vi "Get EST Lib Version from Bitfile.vi"(8 "error in (no error)":errorcluster, 11 "vi info":T2 {"RegisterMap"."Address" format="%.0x"}) -> (0 "error out":errorcluster, 1 "valid bitfile":bool, 2 "EST version enum":T1, 3 "vi info dup":T2 {"RegisterMap"."Address" format="%.0x"}, 5 "EST version string":string)   [LabVIEW 2020, in "Engine Simulation Toolkit System Explorer.lvlib"]
uses:
  Engine Simulation Toolkit System Explorer.lvlib
  <vilib>/rvi/Bitfile/niFpgaBitfileStructure_VI.ctl
  <vilib>/rvi/Bitfile/nirviControlStructure.ctl
  <vilib>/rvi/Bitfile/nirviTypdefDescription.ctl
  <vilib>/rvi/Bitfile/nirviMechanicalAction.ctl
  <vilib>/rvi/Bitfile/nirviSubControlStructure.ctl
  <vilib>/rvi/Bitfile/nirviClusterElementControl.ctl
  <vilib>/picture/picture.llb/imagedata.ctl
  Shared/Bitfile EST Version.ctl
  <vilib>/Utility/Data Type/NI_Data Type.lvlib
  Shared/Engine Simulation Toolkit Shared.lvlib
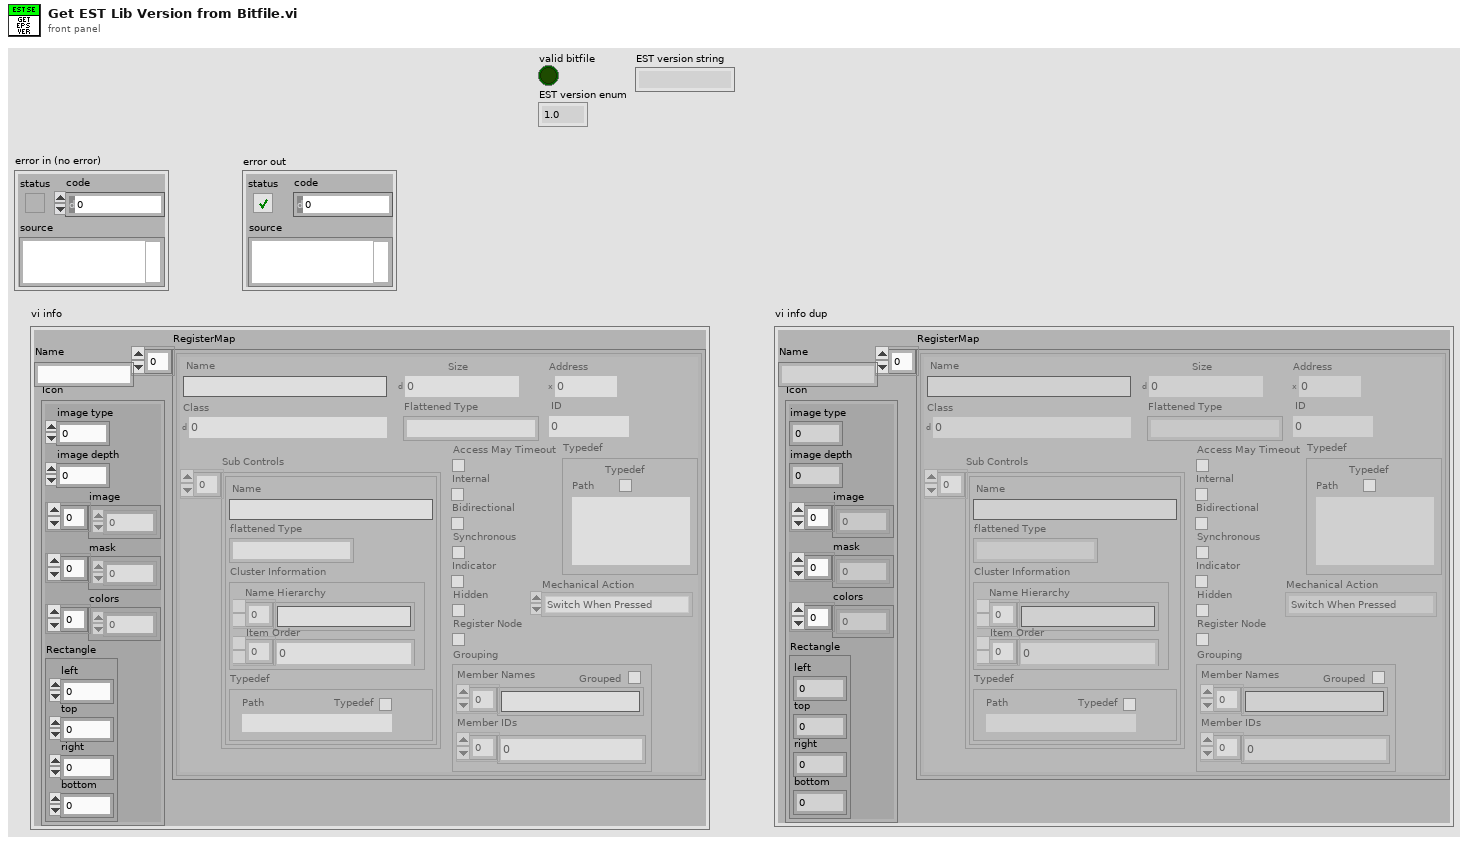
[diagram p1: front panel]
types:
  T1 = typedef "Engine Simulation Toolkit Shared.lvlib/Bitfile EST Version.ctl" = enum16{"1.0", "1.1", "1.2", "1.3", "1.4"}
  T2 = typedef "niFpgaBitfileStructure_VI.ctl" = cluster{"Name":string, "RegisterMap":T3[], "Icon":T8}
  T3 = typedef "nirviControlStructure.ctl" = cluster{"Name":string, "Hidden":bool, "Indicator":bool, "Flattened Type":string, "Grouping":cluster{"Grouped":bool, "Member Names":string[], "Member IDs":u32[]}, "Address":u32, "Size":u32, "Class":u32, "Internal":bool, "Typedef":T4, "ID":u32, "Bidirectional":bool, "Synchronous":bool, "Mechanical Action":T5, "Sub Controls":T6[], "Access May Timeout":bool, "Register Node":bool}
  T4 = typedef "nirviTypdefDescription.ctl" = cluster{"Typedef":bool, "Path":path}
  T5 = typedef "nirviMechanicalAction.ctl" = enum8{"Switch When Pressed", "Switch When Released", "Switch Until Released", "Latch When Pressed", "Latch When Released", "Latch Until Released"}
  T6 = typedef "nirviSubControlStructure.ctl" = cluster{"Name":string, "flattened Type":string, "Cluster Information":T7, "Typedef":T4}
  T7 = typedef "nirviClusterElementControl.ctl" = cluster{"Name Hierarchy":string[], "Item Order":u32[]}
  T8 = typedef "imagedata.ctl" = cluster{"image type":i32, "image depth":i32, "image":u8[], "mask":u8[], "colors":u32[], "Rectangle":cluster{"left":i16, "top":i16, "right":i16, "bottom":i16}}
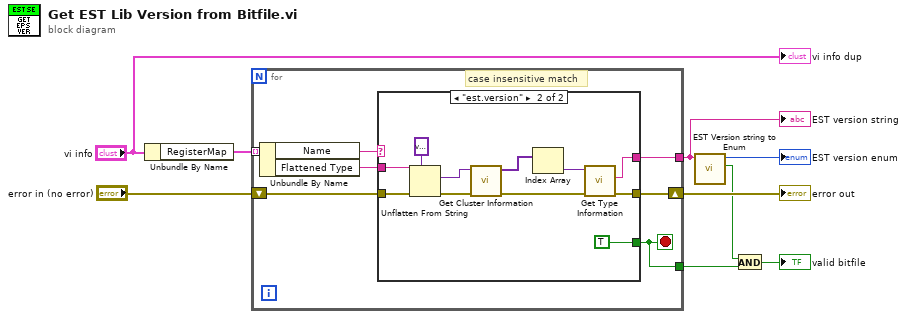
[diagram p0: block diagram]
diagram:
  n1 = Unbundle By Name("vi info") -> ("RegisterMap"=w8:T3[])
  n2 = for {
    shift-right: [w12] -> w7
    shift-left: "error in (no error)" -> [w16]
    tunnel: w8 -> [w15] mode=indexing
    tunnel: [w11] -> w5
    tunnel: [w10] -> w3
    stop <- w11 stop-if-true
    # "case insensitive match"
    n3 = Unbundle By Name(w15) -> ("Name"=w14:string, "Flattened Type"=w13:string)
    n4 = case shown="\"est.version\"" w14 {
      tunnel: w16 -> [w17 w23]
      tunnel: w13 -> [_ w22]
      tunnel: [w17 w25] -> w12
      tunnel: [_ TRUE] -> w11
      tunnel: [_ w18] -> w10
      frame Default {
      }
      frame "est.version" {
        n5 = Unflatten From String(type=variant ("Variant"), binary string=w22, error in (no error)=w23) -> (value=w20:variant, error out=w21:errorcluster)  [unwired: 3 out]
        n6 = call <vilib>:"Get Cluster Information.vi"("error in (no error)"=w21, "variant"=w20) -> ("error out"=w27:errorcluster, "cluster elements"=w28:variant[])  [unwired: 8 in]
        n7 = Index Array(array=w28) -> (element=w26:variant)  [unwired: 1 in]
        n8 = call <vilib>:"Get Type Information.vi"("error in (no error)"=w27, "variant"=w26) -> ("error out"=w25:errorcluster, "name"=w18:string)  [unwired: 5 in, 3 out]
      }
    }
  }
  "error out" <- w7
  "EST version string" <- w3
  n9 = call "EST Version string to Enum.vi"("EST version string"=w3) -> ("valid"=w2:bool, "EST version enum"=→"EST version enum":T1)  [unwired: 9 in]
  n10 = And(x=w2, y=w5) -> (x .and. y?=→"valid bitfile":bool)
  "vi info dup" <- "vi info"
